vi "已连接的设备.vi"() -> ()   [LabVIEW 2013]
panel:
  out "已连接的设备":string[](array[string])
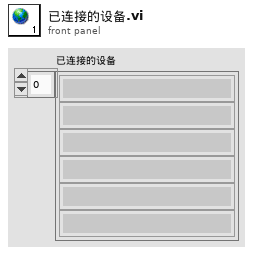
[diagram p1: front panel]
diagram:
